vi "Phasor Correction.vi"(8 "error in (no error)":errorcluster, 9 "system info in":refnum<class "PMU System Info.lvclass">, 10 "timestamps in [s]":dbl[][](array[numeric]), 11 "magnitudes in [RMS]":dbl[][](array[numeric])) -> (0 "error out":errorcluster, 1 "system info out":refnum<class "PMU System Info.lvclass">, 2 "timestamps out [s]":dbl[][](array[numeric]), 3 "magnitudes out [RMS]":dbl[][](array[numeric]))   [LabVIEW 2013, in "NI_EP_PMU.lvlib"]
doc: "Scales the magnitudes of phasors based on the sensitivity of the voltage/current transformer or transducer and compensates the timestamps based on the delays that the data acquisition module, the voltage/current transformer, or the voltage/current transducer introduces."
uses:
  <vilib>/addons/Electrical Power/PMU/NI_EP_PMU.lvlib
  <vilib>/addons/Electrical Power/PMU/Common/Classes/PMU System Info/PMU System Info.lvclass
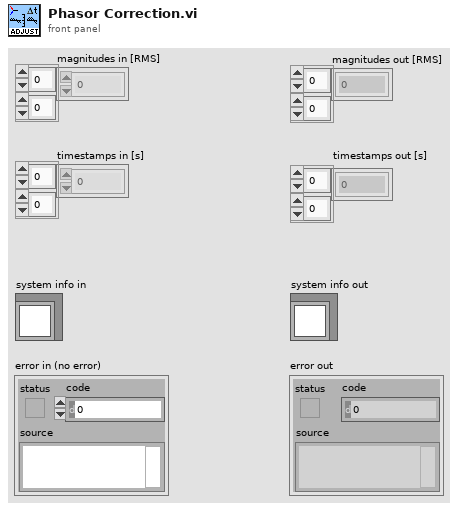
[diagram p1: front panel]
types:
  T1 = typedef "NI_EP_PMU.lvlib/pmu_Physical Channel.ctl" = cluster{"channel phase":T2, "3-phase system ID":u8, "sensor sensitivity":dbl, "sensor group delay [s]":dbl}
  T2 = typedef "NI_EP_PMU.lvlib/pmu_Channel Phase.ctl" = enum16{"Voltage Phase A (L1)", "Voltage Phase B (L2)", "Voltage Phase C (L3)", "Voltage Phase N (Neutral)", "Current Phase A (L1)", "Current Phase B (L2)", "Current Phase C (L3)", "Current Phase N (Neutral)"}
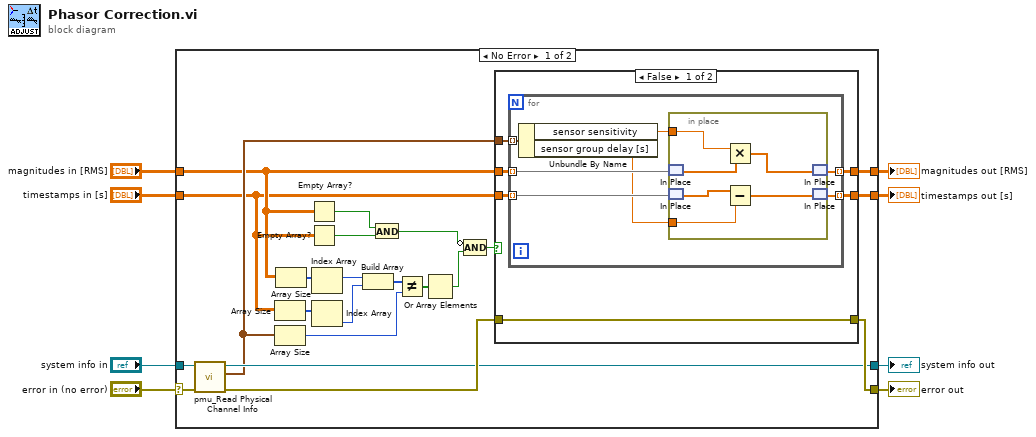
[diagram p0: block diagram]
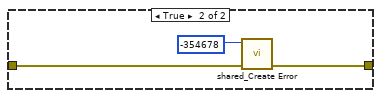
[diagram p2: hidden frame]
diagram:
  n1 = case shown="No Error" "error in (no error)" {
    selector: "error in (no error)" -> [w23 w54]
    tunnel: "system info in" -> [w22 w53]
    tunnel: "timestamps in [s]" -> [w14 _]
    tunnel: "magnitudes in [RMS]" -> [w15 _]
    tunnel: [w29 _] -> w4
    tunnel: [w28 _] -> w3
    tunnel: [w21 w54] -> w2
    tunnel: [w19 w53] -> w1
    frame No Error {
      n2 = call <vilib>:"pmu_Read Physical Channel Info.vi"("error in (no error)"=w23, "system info in"=w22) -> ("error out"=w20:errorcluster, "physical channels"=w18:T1[], "system info out"=w19:refnum<class "PMU System Info.lvclass">)  [unwired: 7 in]
      n3 = Array Size(array=w14) -> (size(s)=w27:i32[])
      n4 = Array Size(array=w18) -> (size(s)=w16:i32)
      n5 = Array Size(array=w15) -> (size(s)=w30:i32[])
      n6 = Empty Array?(array=w15) -> (empty?=w13:bool)
      n7 = Empty Array?(array=w14) -> (empty?=w12:bool)
      n8 = Index Array(array=w30) -> (element=w26:i32)  [unwired: 1 in]
      n9 = Index Array(array=w27) -> (element=w25:i32)  [unwired: 1 in]
      n10 = Build Array(w26, w25) -> (w17:i32[])
      n11 = And(x=w13, y=w12) -> (x .and. y?=w9:bool)
      n12 = Not Equal?(x=w17, y=w16) -> (x != y?=w24:bool[])
      n13 = Or Array Elements(Boolean array=w24) -> (logical OR=w10:bool)
      n14 = Compound Arithmetic op=AND(invert w9, w10) -> (w11:bool)
      n15 = case shown="False" w11 {
        tunnel: w15 -> [w36 _]
        tunnel: w14 -> [w35 _]
        tunnel: [w34 _] -> w29
        tunnel: [w33 _] -> w28
        tunnel: [w32 w50] -> w21
        tunnel: w20 -> [w32 w51]
        tunnel: w18 -> [w31 _]
        frame False {
          n16 = for {
            tunnel: w36 -> [w43] mode=indexing
            tunnel: w35 -> [w42] mode=indexing
            tunnel: [w41] -> w34 mode=indexing
            tunnel: [w40] -> w33 mode=indexing
            tunnel: w31 -> [w39] mode=indexing
            n17 = Unbundle By Name(w39) -> ("sensor sensitivity"=w38:dbl, "sensor group delay [s]"=w37:dbl)
            n18 = in-place {
              in-place-border: w37 -> [w45]
              in-place-border: w38 -> [w49]
              n19 = in-place-match #1(w43) -> (w48:dbl[])
              n20 = in-place-match #2(w42) -> (w46:dbl[])
              n21 = Multiply(x=w49, y=w48) -> (x*y=w47:dbl[])
              n22 = Subtract(x=w46, y=w45) -> (x-y=w44:dbl[])
              n23 = in-place-match #1(w47) -> (w41:dbl[])
              n24 = in-place-match #2(w44) -> (w40:dbl[])
            }
          }
        }
        frame True {
          n25 = call <vilib>:"shared_Create Error.vi"("error in (no error)"=w51, "error code (0)"=-354678) -> ("error out"=w50:errorcluster)  [unwired: 9 in]
        }
      }
    }
    frame Error {
    }
  }
  "error out" <- w2
  "system info out" <- w1
  "magnitudes out [RMS]" <- w4
  "timestamps out [s]" <- w3
